vi "Telnet_Read.vi"(8 "error in (no error)":errorcluster, 9 "bytes to read (1024)":i32=65536, 11 "connection ID In":refnum<k5>) -> (0 "error out":errorcluster, 2 "string out":string, 3 "connection ID out":refnum<k5>)   [LabVIEW 2018]
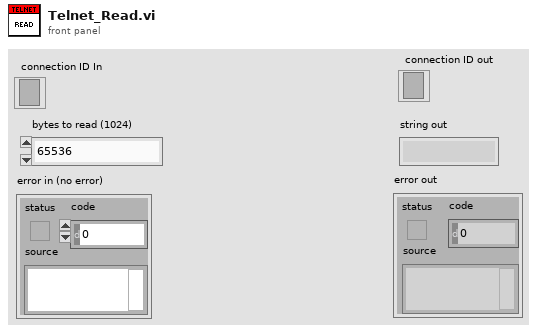
[diagram p1: front panel]
types:
  T1 = enum16{"Standard", "Buffered", "CRLF", "Immediate"}
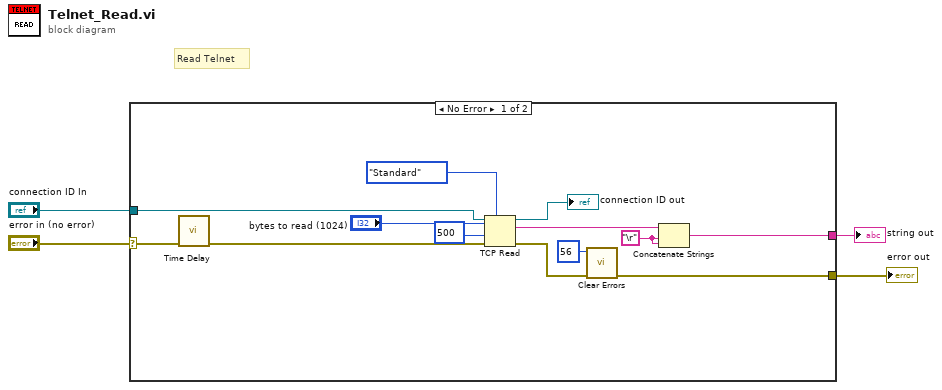
[diagram p0: block diagram]
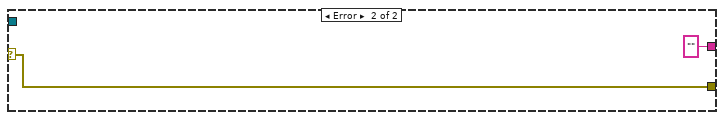
[diagram p2: hidden frame]
diagram:
  # "Read Telnet"
  n1 = case shown="No Error" "error in (no error)" {
    selector: "error in (no error)" -> [w7 w19]
    tunnel: "connection ID In" -> [w12 _]
    tunnel: [w6 ""] -> w2
    tunnel: [w5 w19] -> w1
    frame No Error {
      w8 = "\r"
      n2 = call "Time Delay"("error in (no error)"=w7) -> ("error out"=w10:errorcluster)  [unwired: 10 in]
      n3 = TCP Read(connection ID=w12, bytes to read="bytes to read (1024)", error in (no error)=w10, 7:T1."Standard" ("mode (standard)"), 9:500 ("timeout ms (25000)")) -> (connection ID out=→"connection ID out":refnum<k5>, data out=w9:string, error out=w14:errorcluster)
      n4 = call "Clear Errors.vi"("error in (no error)"=w14, "specific error code to clear (0: all)"=56) -> ("error out"=w5:errorcluster)  [unwired: 4 in, 1 out]
      n5 = Concatenate Strings(w9, w8, w8) -> (w6:string)
    }
    frame Error {
    }
  }
  "string out" <- w2
  "error out" <- w1
